vi "Parameters.vi"(8 "error in (no error)":errorcluster, 11 "Parameterized Test Case In":refnum<class "Parameterized Test Case.lvclass">) -> (0 "error out":errorcluster, 2 "Parameters":T1(array[cluster]))   [LabVIEW 2020, in "Parameterized Test Case.lvclass"]
uses:
  Parameterized Test Case.lvclass
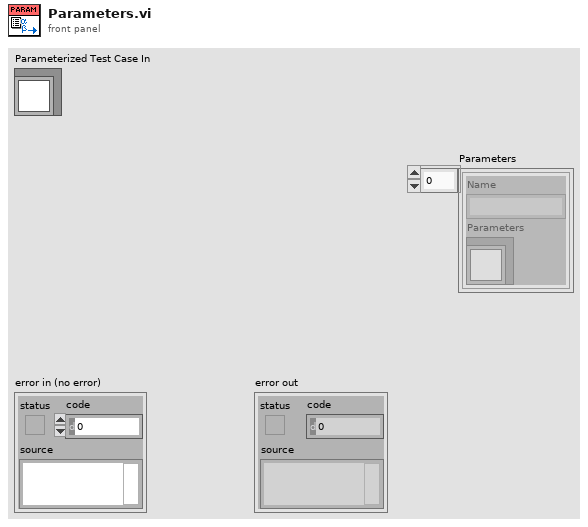
[diagram p1: front panel]
types:
  T1 = cluster{"Name":string, "Parameters":refnum<class "Parameterized Test Case.lvclass">}[]
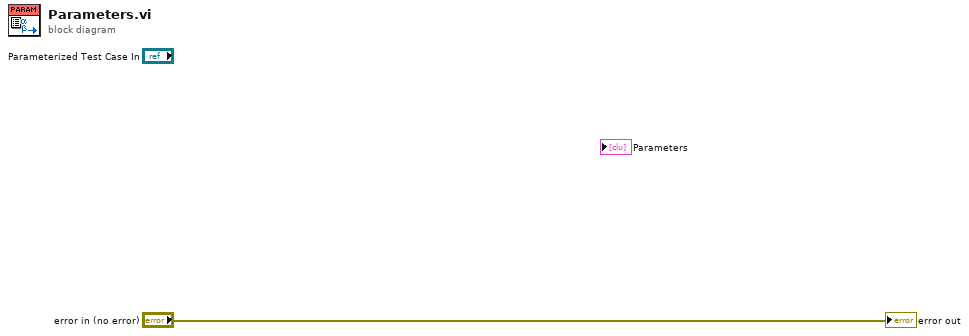
[diagram p0: block diagram]
diagram:
  "error out" <- "error in (no error)"
